vi "TrackerDLL.vi"() -> ()   [LabVIEW 2011]
panel:
  in  "tracker DLL path":path=path "D:/jcnossen1/cudaqi-tracker/cputrack/cputrack_d.dll"
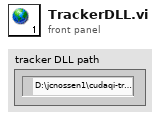
[diagram p1: front panel]
diagram:
